vi "Gamepad Tester.vi"() -> ()   [LabVIEW 2016]
uses:
  <vilib>/Utility/inputDevices.llb/joystickAcquire.vi
  <vilib>/Utility/inputDevices.llb/closeJoystick.vi
panel:
  out "XY Graph":cluster{i32[], i32[]}(graph)
  out "axis info":T1
  in  "stop":bool
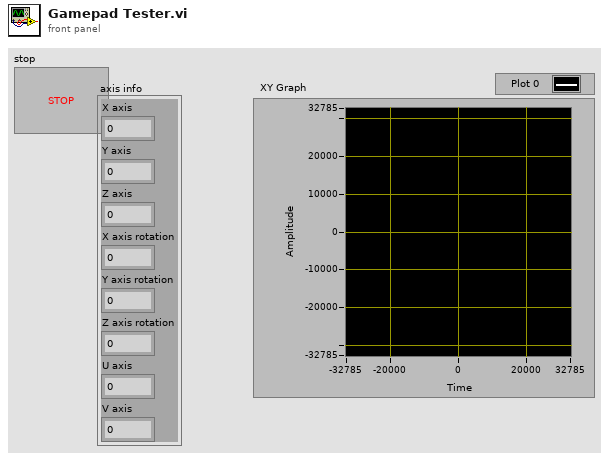
[diagram p1: front panel]
types:
  T1 = cluster{"X axis":i32, "Y axis":i32, "Z axis":i32, "X axis rotation":i32, "Y axis rotation":i32, "Z axis rotation":i32, "U axis":i32, "V axis":i32}
  T2 = cluster{"axes total":u32, "buttons total":u32, "pov total":u32, "device name":string}[]
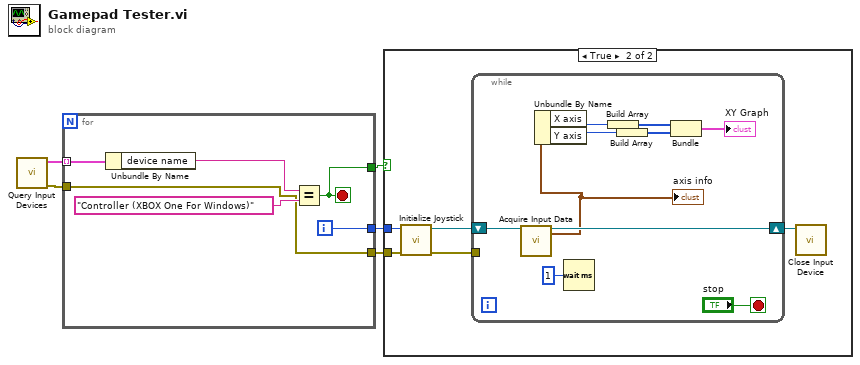
[diagram p0: block diagram]
diagram:
  n1 = call <vilib>:"Query Input Devices.vi"() -> ("error out"=w4:errorcluster, "joystick info"=w5:T2)  [unwired: 8 in, 2 out]
  n2 = for {
    tunnel: w5 -> [w11] mode=indexing
    tunnel: [w8] -> w2
    tunnel: w4 -> [w7]
    tunnel: [w7] -> w3
    tunnel: [w6] -> w1
    i -> [w8]
    stop <- w6 stop-if-true
    n3 = Unbundle By Name(w11) -> ("device name"=w9:string)
    n4 = Equal?(x=w9, y="Controller (XBOX One For Windows)") -> (x = y?=w6:bool)
  }
  n5 = case shown="True" w1 {
    tunnel: w3 -> [_ w13]
    tunnel: w2 -> [_ w12]
    frame False {
    }
    frame True {
      n6 = call <vilib>:"Initialize Joystick.vi"("error in (no error)"=w13, "device index"=w12) -> ("error out"=w14:errorcluster, "device ID"=w16:refnum<k1>)  [unwired: 8 in]
      n7 = while {
        shift-right: [w24] -> w15
        shift-left: w16 -> [w26]
        tunnel: w14 -> [_]
        stop <- "stop" stop-if-true
        n8 = call-poly <vilib>:"Acquire Input Data.vi"("device ID"=w26) -> ("device ID"=w24:refnum<k1>, "axis info"=w22:T1)  [unwired: 14 in, 3 out]
        "axis info" <- w22
        n9 = Unbundle By Name(w22) -> ("X axis"=w21:i32, "Y axis"=w20:i32)
        n10 = Wait (ms)(milliseconds to wait=u32 1) -> ()  [unwired: 1 out]
        n11 = Build Array(w21) -> (w17:i32[])
        n12 = Build Array(w20) -> (w18:i32[])
        n13 = Bundle(w17, w18) -> (→"XY Graph":cluster{i32[], i32[]})  [unwired: 1 in]
      }
      n14 = call-poly <vilib>:"Close Input Device.vi"("device ID"=w15) -> ()  [unwired: 9 in, 1 out]
    }
  }
